vi "Delete Reference.vi"(8 "错误输入（无错误）":errorcluster, 11 "SelfNode*":refnum<data-value>) -> (0 "错误输出":errorcluster)   [LabVIEW 2013, in "PanelRootNode.lvclass"]
uses:
  PanelRootNode.lvclass
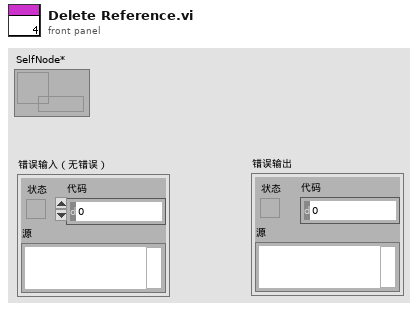
[diagram p1: front panel]
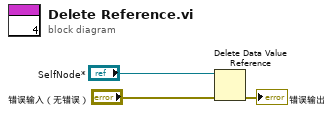
[diagram p0: block diagram]
diagram:
  n1 = Delete Data Value Reference(data value reference="SelfNode*", error in="错误输入（无错误）") -> (error out=→"错误输出":errorcluster)  [unwired: 1 out]
